vi "ferro fit.vi"(7 "ferro response parameters":T1 {"time const b (uS)" scale=0.0..200.0; "amplitude b (V)" scale=0.0..50.0; "time const a (uS)" scale=0.0..200.0; "amplitude a (V)" scale=0.0..50.0}, 11 "time array in (uS)":dbl[](array[numeric])) -> (0 "parameters array out":dbl[](array[numeric]), 2 "voltage array out (V)":dbl[](array[numeric]), 3 "time array out (uS)":dbl[](array[numeric]))   [LabVIEW 2016]
doc: "This subvi recieves the paarmeters of the data and uses a formula to output the voltage array, the same parameters, and the time array for later use.\n\nAlexis Lopez\nP350\nCSUSB Physics"
uses:
  typedefs/ferro response parameter cluster.ctl
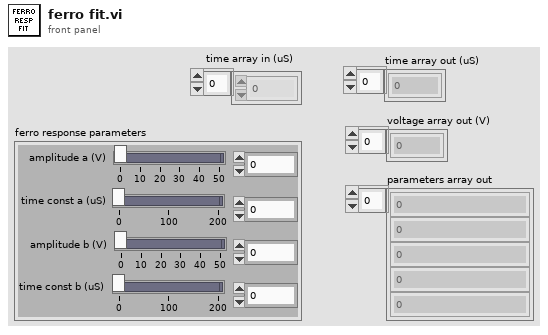
[diagram p1: front panel]
types:
  T1 = typedef "ferro response parameter cluster.ctl" = cluster{"amplitude a (V)":dbl, "time const a (uS)":dbl, "amplitude b (V)":dbl, "time const b (uS)":dbl}
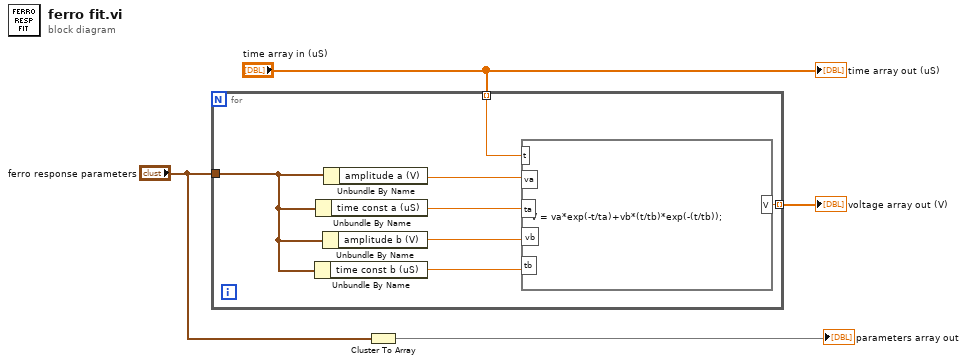
[diagram p0: block diagram]
diagram:
  n1 = for {
    tunnel: [w11] -> w4 mode=indexing
    tunnel: "time array in (uS)" -> [w6] mode=indexing
    tunnel: "ferro response parameters" -> [w5]
    n2 = Unbundle By Name(w5) -> ("time const b (uS)"=w7:dbl)
    n3 = Unbundle By Name(w5) -> ("time const a (uS)"=w9:dbl)
    n4 = Unbundle By Name(w5) -> ("amplitude b (V)"=w8:dbl)
    n5 = Unbundle By Name(w5) -> ("amplitude a (V)"=w10:dbl)
    n6 = formula code="V = va*exp(-t/ta)+vb*(t/tb)*exp(-(t/tb));"("va"=w10, "ta"=w9, "vb"=w8, "tb"=w7, "t"=w6) -> ("V"=w11:dbl)
  }
  "voltage array out (V)" <- w4
  n7 = Cluster To Array(cluster="ferro response parameters") -> (array=→"parameters array out":dbl[])
  "time array out (uS)" <- "time array in (uS)"
